vi "ACQ Summary add+grava.vi"(7 "ACQ full DATA file path":path caption="File path", 8 "summary temp B":u32[][](array[numeric]), 9 "ChipID list 2":u16[](array[numeric]) format="%.0x", 10 "summary temp A":u32[][](array[numeric]), 11 "ChipID list 1":u16[](array[numeric]) format="%.0x") -> ()   [LabVIEW 2015, in "VIPM2.lvlib"]
uses:
  VIPM2.lvlib
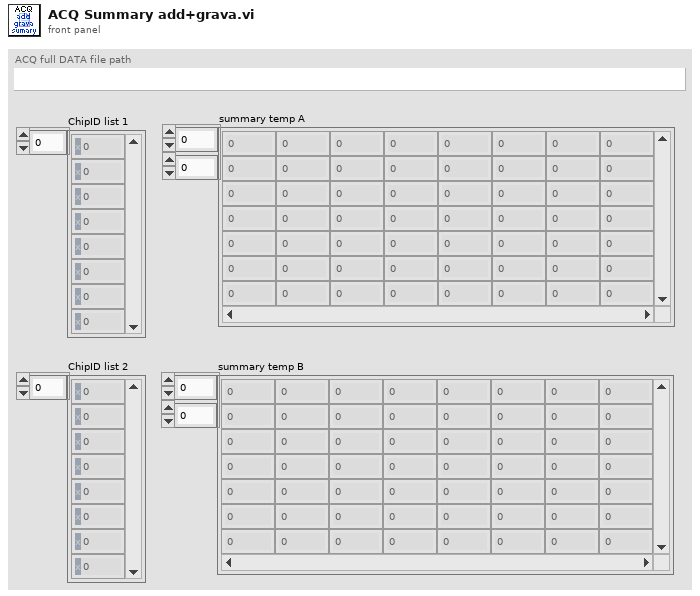
[diagram p1: front panel]
types:
  T1 = enum16{"open", "replace", "create", "open or create", "replace or create", "replace or create with confirmation"}
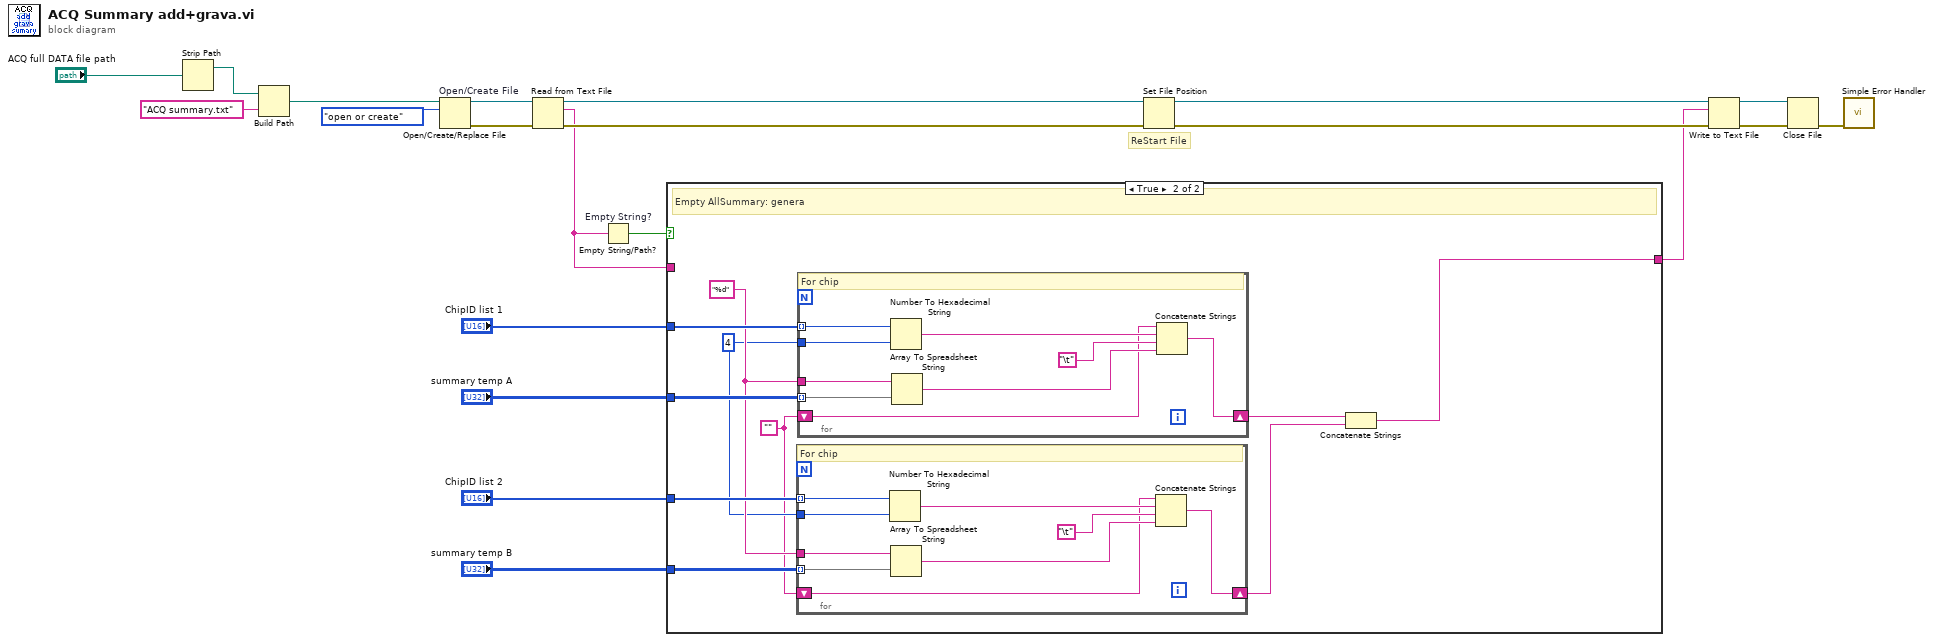
[diagram p0: block diagram]
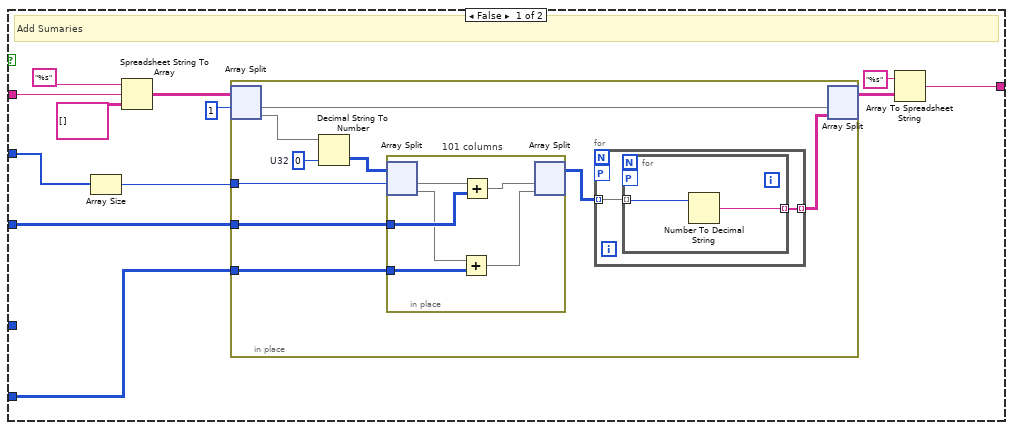
[diagram p2: hidden frame]
diagram:
  # "ReStart File"
  n1 = Strip Path(path="ACQ full DATA file path") -> (stripped path=w19:path)  [unwired: 1 out]
  n2 = Build Path(base path=w19, name or relative path="ACQ summary.txt") -> (appended path=w4:path)
  n3 = Open/Create/Replace File "Open/Create File"(file path (use dialog)=w4, operation (0:open)=T1."open or create") -> (refnum out=w17:refnum<file>, error out=w16:errorcluster)  [unwired: 4 in, 1 out]
  n4 = Read from Text File(file (use dialog)=w17, error in=w16) -> (refnum out=w15:refnum<file>, text=w10:string, error out=w14:errorcluster)  [unwired: 2 in, 1 out]
  n5 = Empty String/Path? "Empty String?"(string/path=w10) -> (empty?=w11:bool)
  n6 = case shown="True" w11 {
    tunnel: w10 -> [w33 _]
    tunnel: "ChipID list 1" -> [w30 w62]
    tunnel: "summary temp A" -> [w28 w61]
    tunnel: "ChipID list 2" -> [_ w59]
    tunnel: "summary temp B" -> [w27 w58]
    tunnel: [w23 w60] -> w5
    frame False {
      # "Add Sumaries"
      n7 = Array Size(array=w30) -> (size(s)=w29:i32)
      n8 = Spreadsheet String To Array(format string="%s", spreadsheet string=w33, array type (2D Dbl)=string[][] []) -> (array=w32:string[][])  [unwired: 1 in]
      n9 = in-place "In Place Element Structure" {
        in-place-border: w29 -> [w41]
        in-place-border: w28 -> [w40]
        in-place-border: w27 -> [w39]
        w37 = u32 0  # U32
        n10 = in-place-split #1(w32, 1) -> (w42:string[][], w38:string[][])
        n11 = Decimal String To Number(string=w38, default (0L)=w37) -> (number=w36:u32[][])  [unwired: 1 in, 1 out]
        n12 = in-place "101 columns" {
          in-place-border: w40 -> [w51]
          in-place-border: w39 -> [w49]
          n13 = in-place-split #2(w36, w41) -> (w52:u32[][], w48:u32[][])
          n14 = Add(x=w48, y=w49) -> (x+y=w47:u32[][])
          n15 = Add(x=w52, y=w51) -> (x+y=w50:u32[][])
          n16 = in-place-split #2(w50, w47) -> (w35:u32[][])  [unwired: 1 out]
        }
        n17 = for {
          tunnel: w35 -> [w44] mode=indexing
          tunnel: [w43] -> w34 mode=indexing
          workers-P: _ -> [_]
          n18 = for {
            tunnel: w44 -> [w46] mode=indexing
            tunnel: [w45] -> w43 mode=indexing
            workers-P: _ -> [_]
            n19 = Number To Decimal String(number=w46) -> (decimal integer string=w45:string)  [unwired: 1 in]
          }
        }
        n20 = in-place-split #1(w42, w34) -> (w24:string[][])  [unwired: 1 out]
      }
      n21 = Array To Spreadsheet String(array=w24, 3:"%s" ("format string")) -> (spreadsheet string=w23:string)  [unwired: 1 in]
    }
    frame True {
      w54 = ""
      w57 = "%d" ("format string")
      w56 = i16 4 ("width (-)")
      # "Empty AllSummary: genera"
      n22 = for {
        tunnel: w59 -> [w71] mode=indexing
        tunnel: w56 -> [w70]
        tunnel: w57 -> [w69]
        tunnel: w58 -> [w68] mode=indexing
        shift-right: [w63] -> w53
        shift-left: w54 -> [w64]
        # "For chip"
        n23 = Number To Hexadecimal String(1:w70, 2:w71) -> (0:w66:string)
        n24 = Array To Spreadsheet String(array=w68, 3:w69) -> (spreadsheet string=w67:string)  [unwired: 1 in]
        n25 = Concatenate Strings "Concatenate Strings"(w64, w66, "\t", w67) -> (w63:string)
      }
      n26 = for {
        tunnel: w62 -> [w80] mode=indexing
        tunnel: w56 -> [w79]
        tunnel: w57 -> [w78]
        tunnel: w61 -> [w77] mode=indexing
        shift-right: [w72] -> w55
        shift-left: w54 -> [w73]
        # "For chip"
        n27 = Number To Hexadecimal String(1:w79, 2:w80) -> (0:w75:string)
        n28 = Array To Spreadsheet String(array=w77, 3:w78) -> (spreadsheet string=w76:string)  [unwired: 1 in]
        n29 = Concatenate Strings "Concatenate Strings"(w73, w75, "\t", w76) -> (w72:string)
      }
      n30 = Concatenate Strings "Concatenate Strings"(w55, w53) -> (w60:string)
    }
  }
  n31 = Set File Position(refnum=w15, error in=w14) -> (refnum out=w13:refnum<file>, error out=w12:errorcluster)  [unwired: 2 in]
  n32 = Write to Text File(file (use dialog)=w13, text=w5, error in=w12) -> (refnum out=w2:refnum<file>, error out=w3:errorcluster)  [unwired: 1 in, 1 out]
  n33 = Close File(refnum=w2, error in=w3) -> (error out=w1:errorcluster)  [unwired: 1 out]
  n34 = call <vilib>:"Simple Error Handler.vi"("error in (no error)"=w1) -> ()  [unwired: 4 in, 5 out]
